vi "ring char motors.vi"(8 "error in":errorcluster, 11 "IOC":string="motors") -> (0 "error out":errorcluster, 2 "Strings And Values Device":cluster{"String":string, "Value":u16}[](array[cluster]), 3 "Strings And Values Card":cluster{"String":string, "Value":u16}[](array[cluster]))   [LabVIEW 2022 SP3]
uses:
  pectus/global/global IOC database.vi
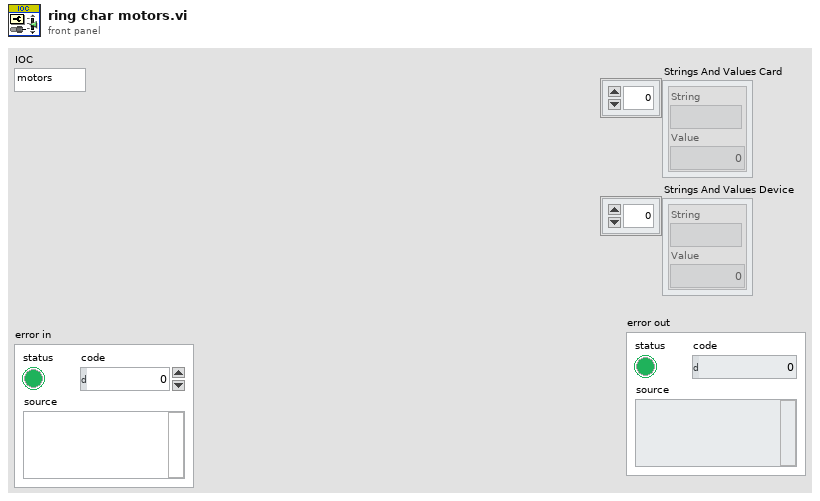
[diagram p1: front panel]
types:
  T1 = typedef "epics database.ctl" = cluster{"IOC":string, "db":string, "Field Values":string[], "Values":string[][], "Type":string, "Card":u16, "Num Dev":u16}
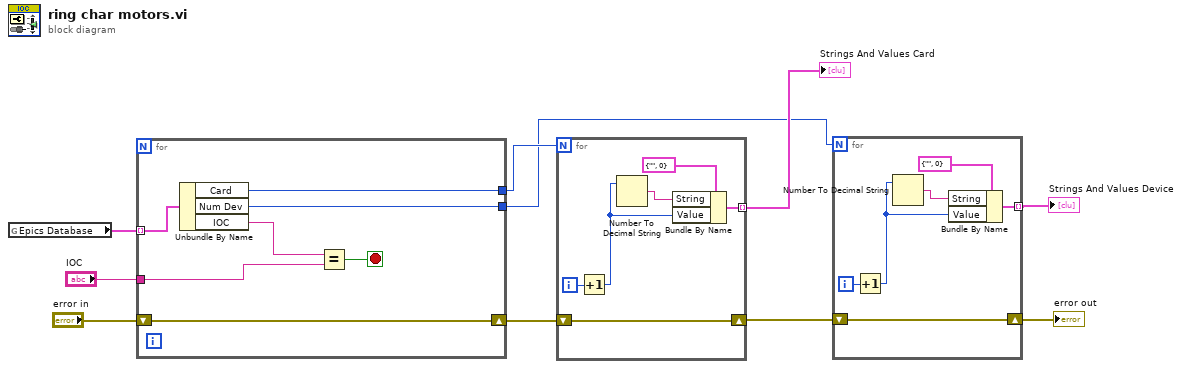
[diagram p0: block diagram]
diagram:
  n1 = global read "global IOC database.vi" "Epics Database"() -> (w10:T1[])
  n2 = for {
    tunnel: w10 -> [w17] mode=indexing
    tunnel: "IOC" -> [w15]
    shift-right: [w14] -> w7
    shift-left: "error in" -> [w14]
    tunnel: [w12] -> w6
    tunnel: [w11] -> w3
    stop <- w13 stop-if-true
    n3 = Unbundle By Name(w17) -> ("Card"=w12:u16, "Num Dev"=w11:u16, "IOC"=w16:string)
    n4 = Equal?(x=w16, y=w15) -> (x = y?=w13:bool)
  }
  n5 = for {
    N: w6 -> [_]
    shift-right: [w23] -> w4
    shift-left: w7 -> [w23]
    tunnel: [w22] -> w5 mode=indexing
    i -> [w20]
    n6 = Increment(x=w20) -> (x+1=w18:i32)
    n7 = Number To Decimal String(number=w18) -> (decimal integer string=w19:string)  [unwired: 1 in]
    n8 = Bundle By Name(cluster=cluster{"String":string, "Value":u16} {"String"="", "Value"=0}, "String"=w19, "Value"=w18) -> (w22:cluster{"String":string, "Value":u16})
  }
  "Strings And Values Card" <- w5
  n9 = for {
    N: w3 -> [_]
    shift-right: [w29] -> w2
    shift-left: w4 -> [w29]
    tunnel: [w28] -> w1 mode=indexing
    i -> [w26]
    n10 = Increment(x=w26) -> (x+1=w24:i32)
    n11 = Number To Decimal String(number=w24) -> (decimal integer string=w25:string)  [unwired: 1 in]
    n12 = Bundle By Name(cluster=cluster{"String":string, "Value":u16} {"String"="", "Value"=0}, "String"=w25, "Value"=w24) -> (w28:cluster{"String":string, "Value":u16})
  }
  "error out" <- w2
  "Strings And Values Device" <- w1
